vi "Initialize.vi"(8 "error in (no error)":errorcluster, 9 "Requestor":string, 10 "Requestee":string, 11 "Red Pitaya in":refnum<class "Red Pitaya.lvclass">) -> (0 "error out":errorcluster, 3 "Red Pitaya out":refnum<class "Red Pitaya.lvclass">)   [LabVIEW 2015, in "Red Pitaya.lvclass"]
uses:
  Red Pitaya.lvclass
  NHMFL_Core/Libraries/Red Pitaya/RP Command.ctl
  Mag Lab Measure/Hardware/Spectrum Analyzer/Spectrum Analyzer.lvclass/Spectrum Analyzer.ctl
  Red Pitaya.lvclass/Red Pitaya.ctl
  Mag Lab Measure/Hardware/Spectrum Analyzer/Read Frequencies.vi
  Mag Lab Measure/Hardware/Spectrum Analyzer/Read Duration.vi
  Mag Lab Measure/Hardware/Spectrum Analyzer/Spectrum Analyzer.lvclass
  Mag Lab Measure/Mag Lab Error Handler/Mag Lab Error Handler.lvclass
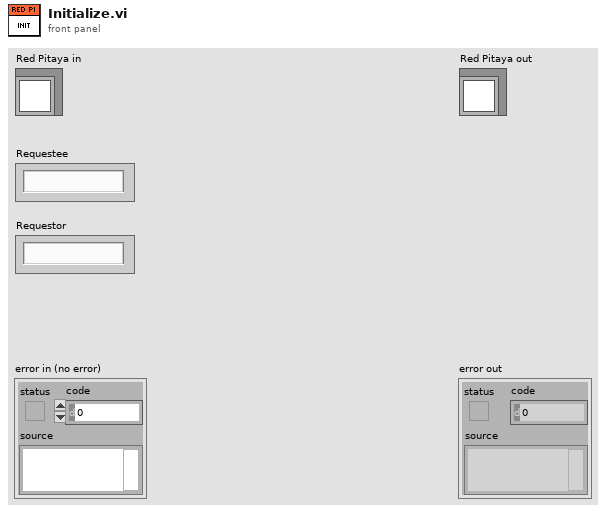
[diagram p1: front panel]
types:
  T1 = typedef "RP Command.ctl" = enum16{"Set frequency", "Read IDN", "Stop server", "Get status", "Get temperature", "Connect client", "Arm", "Software trigger", "Get whole buffer", "Get chunk", "System call", "Get config", "Set config", "Read FIFO", "Play pattern", "Set frequency batch"}
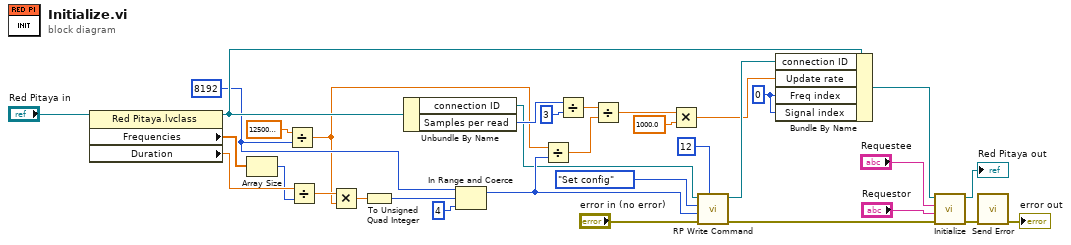
[diagram p0: block diagram]
diagram:
  w8 = 0 ("Freq index")
  w23 = u64 8192 ("x")
  n1 = property class="Red Pitaya.lvclass"(reference="Red Pitaya in") -> (reference out=w24:refnum<class "Red Pitaya.lvclass">, "Frequencies"=w29:dbl[], "Duration"=w7:dbl)  [unwired: 1 in, 1 out]
  n2 = Array Size(array=w29) -> (size(s)=w6:i32)
  n3 = Divide(x=125000000.0 ("y"), y=w23) -> (x/y=w13:dbl)
  n4 = Divide(x=w7, y=w6) -> (x/y=w27:dbl)
  n5 = Multiply(x=w27, y=w13) -> (x*y=w26:dbl)
  n6 = To Unsigned Quad Integer(1:w26) -> (0:w12:u64)
  n7 = Unbundle By Name(w24) -> ("connection ID"=w2:refnum<k5>, "Samples per read"=w15:i32)
  n8 = In Range and Coerce(upper limit=w23, x=w12, lower limit=u64 4 ("Command payload")) -> (coerced(x)=w5:u64)  [unwired: 1 out]
  n9 = Divide(x=w13, y=w5) -> (x/y=w10:dbl)
  n10 = Divide(x=w15, y=3) -> (x/y=w11:dbl)
  n11 = Divide(x=w11, y=w10) -> (x/y=w9:dbl)
  n12 = Multiply(x=w9, y=1000.0) -> (x*y=w4:dbl)
  n13 = call "RP Write Command.vi"("Config offset"=u64 12, "Error In"="error in (no error)", "Command payload"=w5, "Command number"=RP_Command."Set config", "connection ID"=w2) -> ("Error Out"=w20:errorcluster, "connection ID out"=w16:refnum<k5>)  [unwired: 4 in, 1 out]
  n14 = Bundle By Name(cluster=w24, "connection ID"=w16, "Update rate"=w4, "Freq index"=w8, "Signal index"=w8) -> (w17:refnum<class "Red Pitaya.lvclass">)
  n15 = call-parent "Initialize.vi"("error in (no error)"=w20, "Requestor"="Requestor", "Requestee"="Requestee", "Mag Lab Root in"=w17) -> ("error out"=w19:errorcluster, "Mag Lab Root out"=→"Red Pitaya out":refnum<class "Red Pitaya.lvclass">)  [unwired: 6 in]
  n16 = call "Send Error.vi"("error in (no error)"=w19) -> ("error out"=→"error out":errorcluster)  [unwired: 9 in, 1 out]
